vi "CVT Bool IndexRead.vi"(3 "error in (no error)":errorcluster, 5 "Tag Index":i32) -> (0 "error out":errorcluster, 1 "Value":bool)   [LabVIEW 2010]
uses:
  Current Value Table.lvlib
  DataTypes/Boolean_Read Index.vi
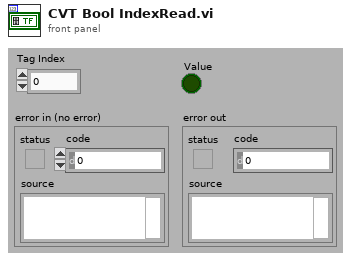
[diagram p1: front panel]
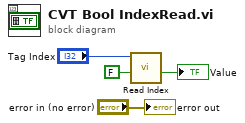
[diagram p0: block diagram]
diagram:
  n1 = call-poly "Read Index.vi"("Default"=FALSE, "Index"="Tag Index") -> ("Value"=→"Value":bool)  [unwired: 9 in]
  "error out" <- "error in (no error)"
